vi "CohortDetailedWaveforms.vi"(0 "Cohort in":refnum<class "Cohort.lvclass">, 1 "Sampling Frequency [Hz]":u32=100000 format="%.2p", 3 "error in (no error)":errorcluster) -> (7 "Cohort out":refnum<class "Cohort.lvclass">, 10 "error out":errorcluster)   [LabVIEW 2012, in "Cohort.lvclass"]
uses:
  Cohort.lvclass
  Electrode.lvclass
  CohortEleWfmPanel.ctl
  StimulCtrls.lvlib
panel:
  in  "Reload":bool
  in  "Close Panel":bool
  out "Individual Electrode Waveforms":T1
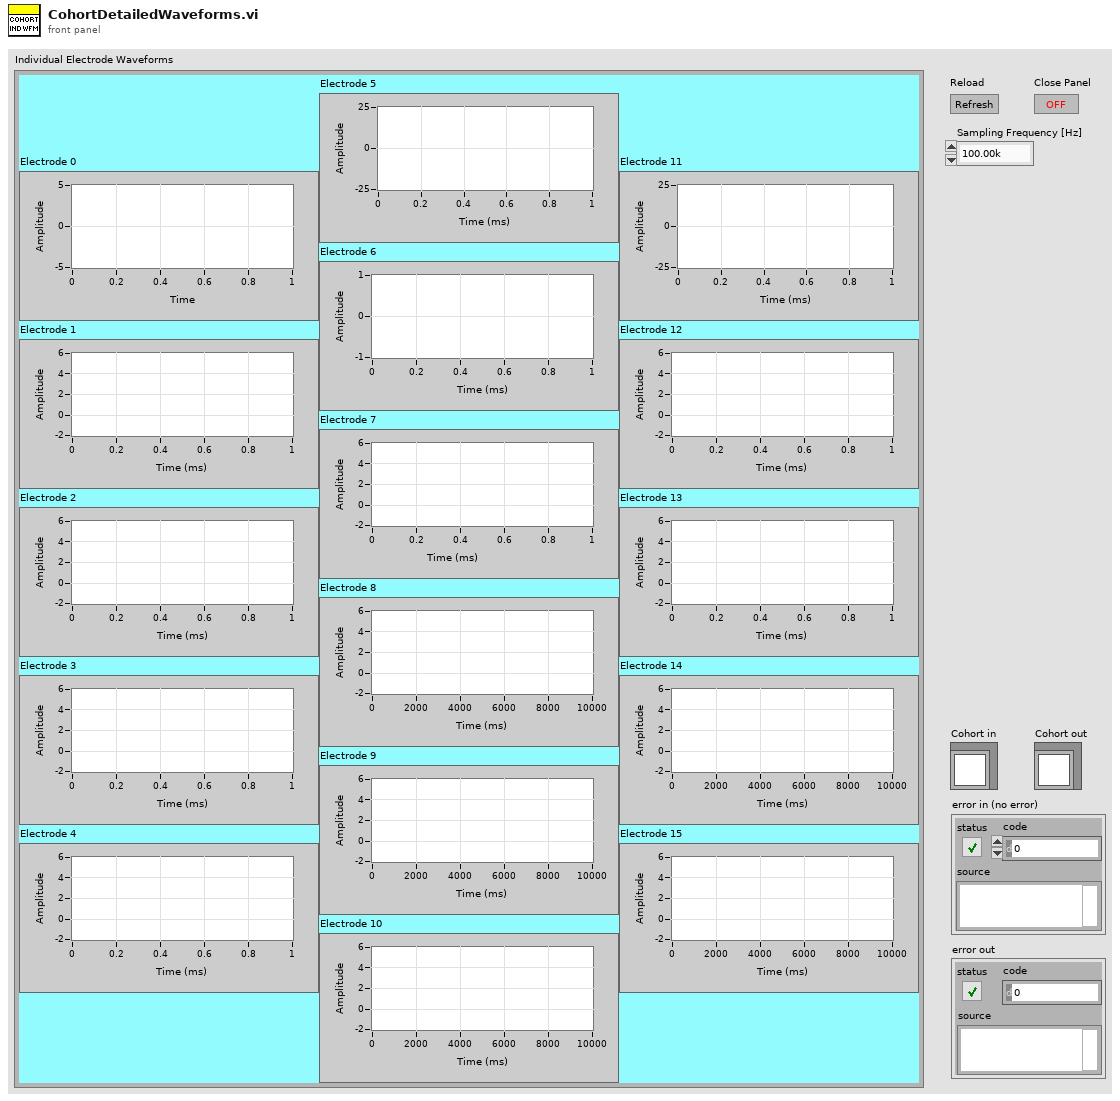
[diagram p1: front panel]
types:
  T1 = typedef "StimulCtrls.lvlib/CohortEleWfmPanel.ctl" = cluster{"Electrode 0":waveform(dbl), "Electrode 1":waveform(dbl), "Electrode 2":waveform(dbl), "Electrode 3":waveform(dbl), "Electrode 4":waveform(dbl), "Electrode 5":waveform(dbl), "Electrode 6":waveform(dbl), "Electrode 7":waveform(dbl), "Electrode 8":waveform(dbl), "Electrode 9":waveform(dbl), "Electrode 10":waveform(dbl), "Electrode 11":waveform(dbl), "Electrode 12":waveform(dbl), "Electrode 13":waveform(dbl), "Electrode 14":waveform(dbl), "Electrode 15":waveform(dbl)}
  T2 = enum32{"Invalid", "Standard", "Closed", "Hidden", "Minimized", "Maximized"}
  T3 = cluster{"[0]":waveform(dbl), "[1]":waveform(dbl), "[2]":waveform(dbl), "[3]":waveform(dbl), "[4]":waveform(dbl), "[5]":waveform(dbl), "[6]":waveform(dbl), "[7]":waveform(dbl), "[8]":waveform(dbl), "[9]":waveform(dbl), "[10]":waveform(dbl), "[11]":waveform(dbl), "[12]":waveform(dbl), "[13]":waveform(dbl), "[14]":waveform(dbl), "[15]":waveform(dbl)}
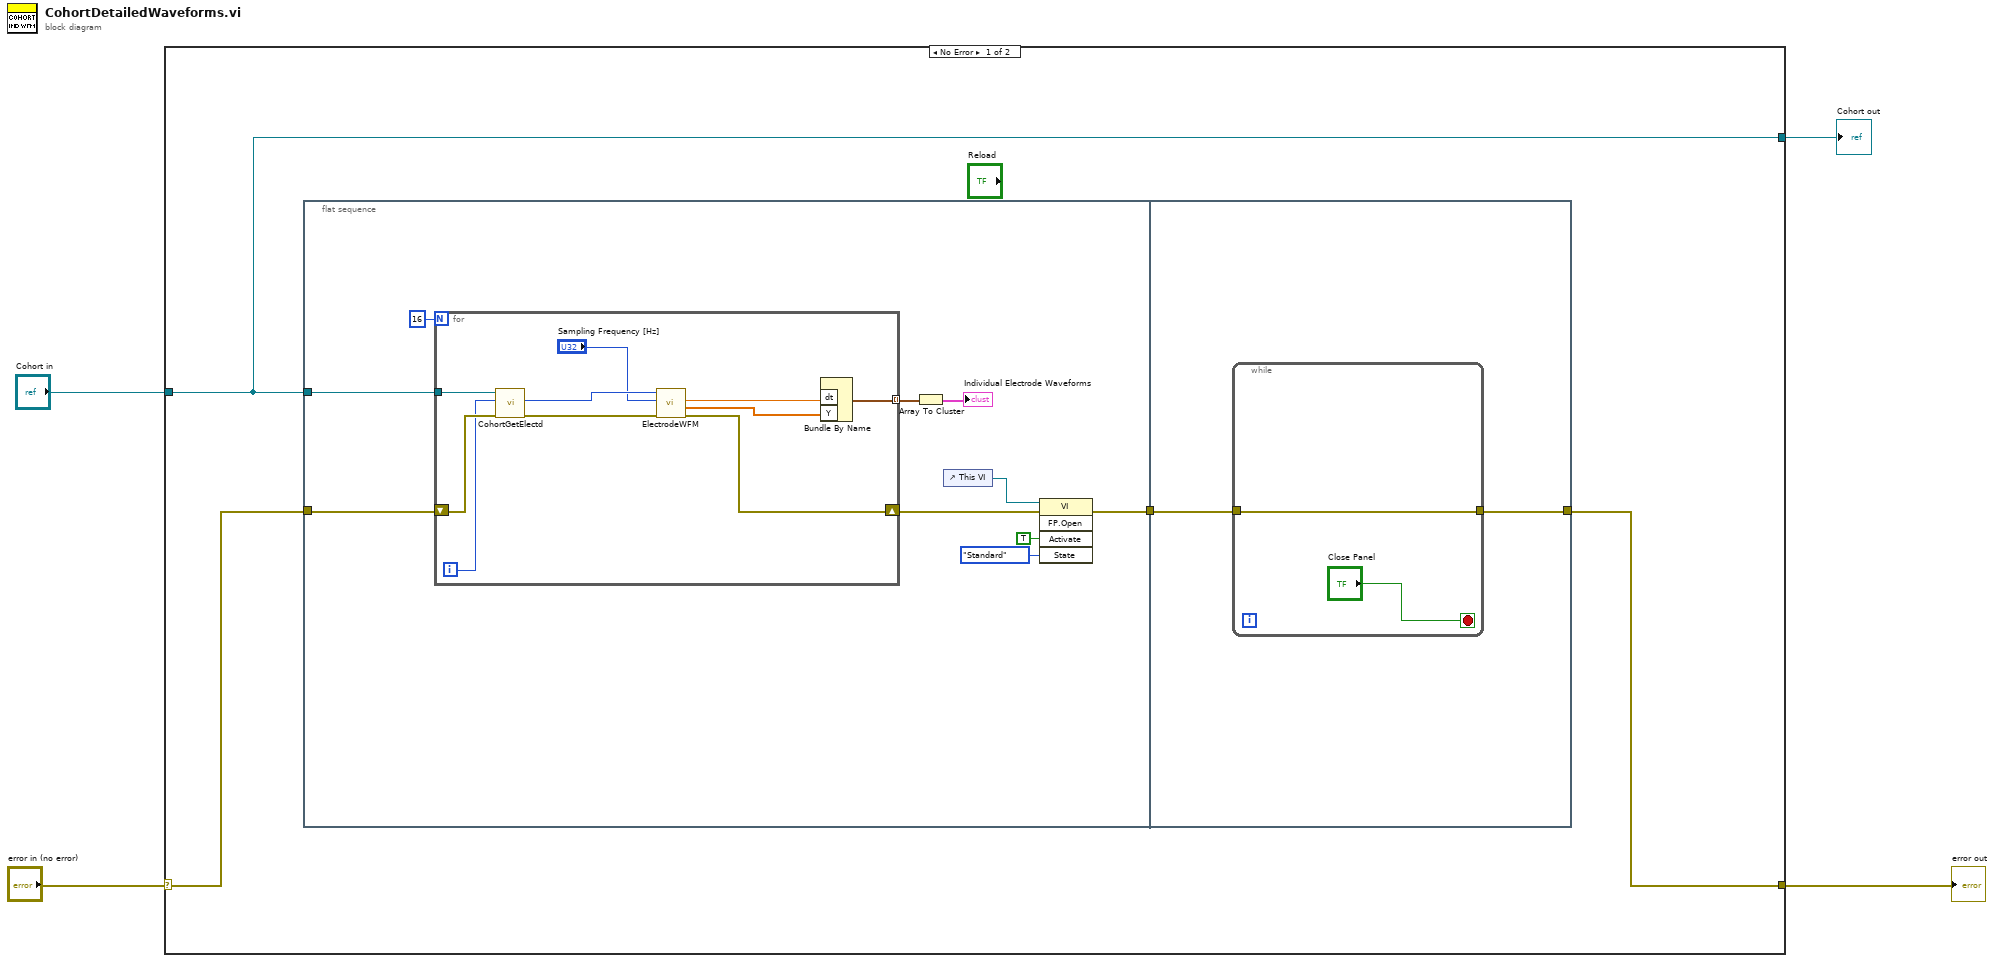
[diagram p0: block diagram]
diagram:
  n1 = case shown="No Error" "error in (no error)" {
    selector: "error in (no error)" -> [w8 w34]
    tunnel: [w5 w34] -> w1
    tunnel: "Cohort in" -> [w6 w33]
    tunnel: [w6 w33] -> w2
    frame No Error {
      n2 = flat-sequence {
        tunnel: w6 -> [w13]
        tunnel: w8 -> [w12]
        tunnel: [w10] -> w7
        tunnel: w7 -> [w30]
        tunnel: [w29] -> w5
        frame #0 {
          n3 = for {
            N: 16 -> [_]
            tunnel: [w28] -> w15 mode=indexing
            tunnel: w13 -> [w27]
            shift-right: [w21] -> w11
            shift-left: w12 -> [w20]
            i -> [w19]
            n4 = call-dynamic "CohortGetElectd.vi"("error in (no error)"=w20, 10:w19, "Cohort in"=w27) -> ("error out"=w25:errorcluster, "Pulse Frequency [Hz]"=w26:u8)  [unwired: 5 in, 2 out]
            n5 = call "ElectrodeWFM.vi"("Electrode in"=w26, "Sampling Rate [Hz]"="Sampling Frequency [Hz]", "error in (no error)"=w25) -> ("dt [s]"=w23:dbl, "Signal Array"=w22:dbl[], "error out"=w21:errorcluster)  [unwired: 3 in, 2 out]
            n6 = Bundle By Name("dt"=w23, "Y"=w22) -> (w28:waveform(dbl))  [unwired: 1 in]
          }
          n7 = Array To Cluster(array=w15) -> (cluster=→"Individual Electrode Waveforms":T3)
          n8 = control-ref of="This VI"() -> (w18:refnum<vi>)
          n9 = invoke class="VI" method="FP.Open"(reference=w18, error in=w11, "Activate"=TRUE ("Activate?"), "State"=T2."Standard") -> (error out=w10:errorcluster)  [unwired: 1 in, 4 out]
        }
        frame #1 {
          n10 = while {
            tunnel: w30 -> [w31]
            tunnel: [w31] -> w29
            stop <- "Close Panel" stop-if-true
          }
        }
      }
    }
    frame Error {
    }
  }
  "error out" <- w1
  "Cohort out" <- w2
